vi "Part 1 Array Size, Index Array.vi"() -> ()   [LabVIEW 2020]
panel:
  out "element":dbl
  out "size(s)":i32
  in  "array":dbl[](array[numeric])
  # "Part 1"
  # "Array Size & Index Array"
  # "0          1        2         3"
  # "3"
  # "1"
  # "2"
  # "4"
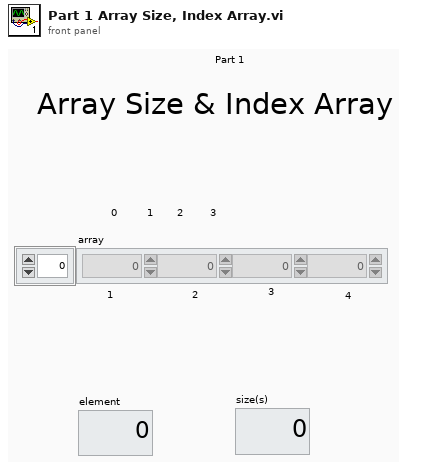
[diagram p1: front panel]
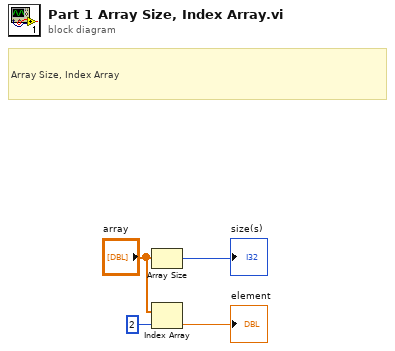
[diagram p0: block diagram]
diagram:
  # "Array Size, Index Array"
  n1 = Array Size(array="array") -> (size(s)=→"size(s)":i32)
  n2 = Index Array "Index Array"(array="array", index=2) -> (element=→"element":dbl)
